vi "initConversion.vi"(0 "phCam":u64, 11 "error in (no error)":errorcluster) -> (4 "ph out":u64, 6 "phConv":u64, 8 "colorPattern":u16, 13 "yOffset":u16, 14 "xOffset":u16, 15 "error out":errorcluster)   [LabVIEW 2020]
uses:
  ImageInformation.lvlib
  Convert.lvlib
  CameraDescription.lvlib
  GeneralCameraStatus.lvlib
  ImageSensor.lvlib
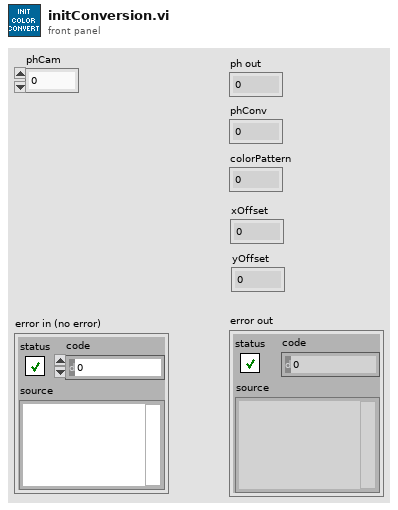
[diagram p1: front panel]
types:
  T1 = cluster{"wCamType":u16, "wCamSubType":u16, "dwSerialNumber":u32, "dwHWVersion":u32, "dwFWVersion":u32, "InterfaceType":u16, "PCO_FW_Vers":cluster{"wDeviceNum":u16, "PCO_SC2_Firmware_DESC":cluster{"szName":string, "bMinorRev":u8, "bMajorRev":u8, "wVariant":u16}[]}, "PCO_HW_Vers":cluster{"wBoardNum":u16, "PCO_SC2_Hardware_DESC":cluster{"szName":string, "wBatchNo":u16, "wRevision":u16, "wVariant":u16}[]}}
  T2 = cluster{"wSensorTypeDESC":u16, "wSensorSubTypeDESC":u16, "wMaxHorzResStdDESC":u16, "wMaxVertResStdDESC":u16, "wMaxHorzResExtDESC":u16, "wMaxVertResExtDESC":u16, "wDynResDESC":u16, "wMaxBinHorzDESC":u16, "wBinHorzSteppingDESC":u16, "wMaxBinVertDESC":u16, "wBinVertSteppingDESC":u16, "wRoiHorStepsDESC":u16, "wRoiVertStepsDESC":u16, "wNumADCsDESC":u16, "wMinSizeHorzDESC":u16, "dwPixelRateDESC":u32[], "wConvFactDESC":u16[], "sCoolingSetpoints":i16[], "wSoftRoiHorStepsDESC":u16, "wSoftRoiVertStepsDESC":u16, "wIRDESC":u16, "wMinSizeVertDESC":u16, "dwMinDelayDESC":u32, "dwMaxDelayDESC":u32, "dwMinDelayStepDESC":u32, "dwMinExposureDESC":u32, "dwMaxExposureDESC":u32, "dwMinExposureStepDESC":u32, "dwMinDelayIRDESC":u32, "dwMaxDelayIRDESC":u32, "dwMinExposureIRDESC":u32, "dwMaxExposureIRDESC":u32, "wTimeTableDESC":u16, "wDoubleImageDESC":u16, "sMinCoolSetDESC":i16, "sMaxCoolSetDESC":i16, "sDefaultCoolSetDESC":i16, "wPowerDownModeDESC":u16, "wOffsetRegulationDESC":u16, "wColorPatternDESC":u16, "wPatternTypeDESC":u16, "wNumCoolingSetpoints":u16, "dwGeneralCapsDESC1":u32, "dwGeneralCapsDESC2":u32, "dwExtSyncFrequency":u32[], "dwGeneralCapsDESC3":u32, "dwGeneralCapsDESC4":u32}
  T3 = cluster{"iConversionFactor":i32, "iDataBits":i32, "iSensorInfoBits":i32, "iDarkOffset":i32, "strColorCoeff":dbl[], "iCamNum":i32, "hCamera":u64}
  T4 = cluster{"wScale_minmax":u16, "iScale_maxmax":i32, "iScale_min":i32, "iScale_max":i32, "iColor_temp":i32, "iColor_tint":i32, "iColor_saturation":i32, "iColor_vibrance":i32, "iContrast":i32, "iGamma":i32, "iSRGB":i32, "pHistogramData":u64, "dwProcessingFlags":u32, "wProzValue4Min":u16, "wProzValue4Max":u16}
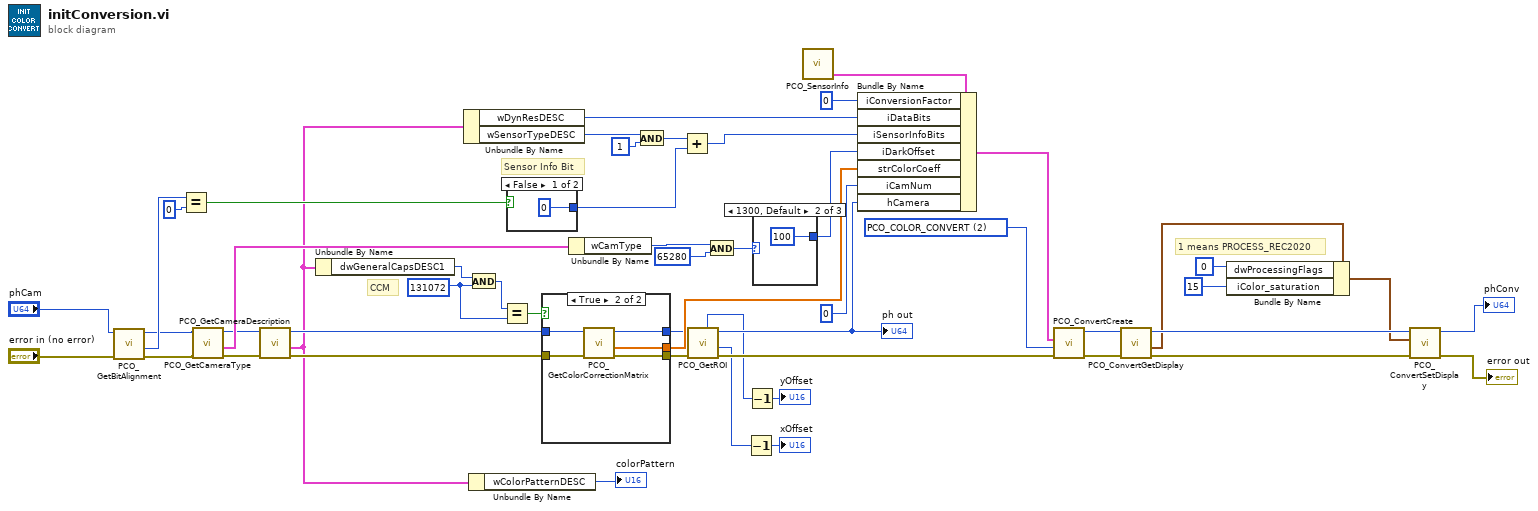
[diagram p0: block diagram]
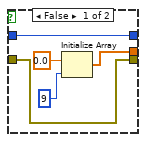
[diagram p2: hidden frame]
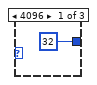
[diagram p3: hidden frame]
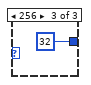
[diagram p4: hidden frame]
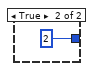
[diagram p5: hidden frame]
diagram:
  w2 = u32 131072 ("y")
  w36 = 2 items=["PCO_BW_CONVERT"=1, "PCO_COLOR_CONVERT"=2, "PCO_PSEUDO_CONVERT"=3, "PCO_COLOR16_CONVERT"=4] ("iConvertType")
  # "CCM"
  # "1 means PROCESS_REC2020"
  # "Sensor Info Bit"
  n1 = call "PCO_GetBitAlignment.vi"("error in (no error)"="error in (no error)", "ph"="phCam") -> ("error out"=w11:errorcluster, "wBitAlignment"=w46:u16, "ph out"=w12:u64)  [unwired: 6 in, 1 out]
  n2 = Equal?(x=w46, y=u16 0) -> (x = y?=w44:bool)
  n3 = call "PCO_GetCameraType.vi"("error in (no error)"=w11, "ph"=w12) -> ("error out"=w9:errorcluster, "strCamType"=w13:T1, "ph out"=w10:u64)  [unwired: 6 in, 1 out]
  n4 = call "PCO_GetCameraDescription.vi"("error in (no error)"=w9, "ph"=w10) -> ("error out"=w8:errorcluster, "strDescription"=w6:T2, "ph out"=w7:u64)  [unwired: 6 in, 1 out]
  n5 = Unbundle By Name(w6) -> ("dwGeneralCapsDESC1"=w5:u32)
  n6 = Unbundle By Name(w6) -> ("wDynResDESC"=w27:u16, "wSensorTypeDESC"=w48:u16)
  n7 = And(x=w5, y=w2) -> (x .and. y?=w3:u32)
  n8 = Unbundle By Name(w6) -> ("wColorPatternDESC"=→"colorPattern":u16)
  n9 = Equal?(x=w3, y=w2) -> (x = y?=w1:bool)
  n10 = case shown="False" w44 {
    tunnel: [u16 0 ("y") u16 2 ("y")] -> w42
    frame False {
    }
    frame True {
    }
  }
  n11 = case shown="True" w1 {
    tunnel: [w55 w64] -> w41
    tunnel: [w59 w63] -> w20
    tunnel: w8 -> [w58 w61]
    tunnel: w7 -> [w59 w62]
    tunnel: [w58 w60] -> w4
    frame False {
      n12 = Initialize Array(0.0 ("element"), 9 ("dimension size")) -> (w55:dbl[])
    }
    frame True {
      n13 = call "PCO_GetColorCorrectionMatrix.vi"("error in (no error)"=w61, "ph"=w62) -> ("error out"=w60:errorcluster, "pdMatrix"=w64:dbl[], "ph out"=w63:u64)  [unwired: 6 in, 1 out]
    }
  }
  n14 = Unbundle By Name(w13) -> ("wCamType"=w39:u16)
  n15 = And(x=w48, y=u16 1) -> (x .and. y?=w43:u16)
  n16 = Add(x=w43, y=w42) -> (x+y=w26:u16)
  n17 = call "PCO_GetROI.vi"("error in (no error)"=w4, "ph"=w20) -> ("error out"=w18:errorcluster, "wRoiX0"=w17:u16, "ph out"=w19:u64, "wRoiY0"=w15:u16)  [unwired: 3 in, 3 out]
  "ph out" <- w19
  n18 = And(x=w39, y=u16 65280) -> (x .and. y?=w38:u16)
  n19 = Decrement(x=w17) -> (x-1=→"xOffset":u16)
  n20 = Decrement(x=w15) -> (x-1=→"yOffset":u16)
  n21 = case shown="1300, Default" w38 {
    tunnel: [32 ("iDarkOffset") 100 ("iDarkOffset") 32 ("iDarkOffset")] -> w37
    frame 4096 {
    }
    frame 4864, Default {
    }
    frame 256 {
    }
  }
  n22 = call "PCO_SensorInfo.vi"() -> ("PCO_SensorInfo"=w28:T3)  [unwired: 4 in, 4 out]
  n23 = Bundle By Name(cluster=w28, "iConversionFactor"=0, "iDataBits"=w27, "iSensorInfoBits"=w26, "iDarkOffset"=w37, "strColorCoeff"=w41, "iCamNum"=0, "hCamera"=w19) -> (w25:T3)
  n24 = call "PCO_ConvertCreate.vi"("error in (no error)"=w18, "iConvertType"=w36, "strSensor"=w25) -> ("error out"=w34:errorcluster, "ph out"=w35:u64)  [unwired: 6 in, 1 out]
  n25 = call "PCO_ConvertGetDisplay.vi"("error in (no error)"=w34, "ph"=w35) -> ("error out"=w33:errorcluster, "strDisplay"=w23:T4, "ph out"=w32:u64)  [unwired: 6 in, 1 out]
  n26 = Bundle By Name(cluster=w23, "dwProcessingFlags"=u32 0, "iColor_saturation"=15) -> (w31:T4)
  n27 = call "PCO_ConvertSetDisplay.vi"("error in (no error)"=w33, "strDisplay"=w31, "ph"=w32) -> ("error out"=→"error out":errorcluster, "ph out"=→"phConv":u64)  [unwired: 6 in, 1 out]
